vi "Write Paragraphe.vi"(8 "error in (no error)":errorcluster, 10 "Paragraphe cluster":T1, 11 "PDF Report Class in":refnum<class "PDF Report Class.lvclass">) -> (0 "error out":errorcluster, 3 "PDF Report Class out":refnum<class "PDF Report Class.lvclass">)   [LabVIEW 2019, in "PDF Report Class.lvclass"]
uses:
  <userlib>/Exaprom PDF/LV Class/PDF Report Class/PDF Report Class.lvclass
  <userlib>/Exaprom PDF/Controls/Initialization Controls/Defaut Paragraphe and Line Spacing.ctl
  <userlib>/Exaprom PDF/Controls/Text Controls/Texte alignement.ctl
  <userlib>/Exaprom PDF/Controls/Text Controls/Line spacing.ctl
  <userlib>/Exaprom PDF/LV Class/PDF Report Class/PDF Report Class.lvclass/PDF Report Class.ctl
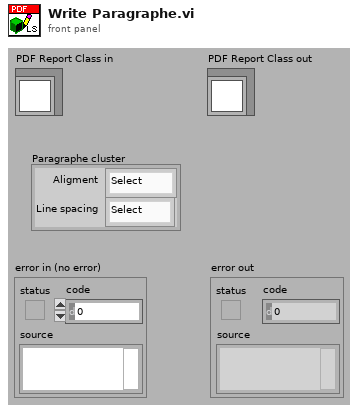
[diagram p1: front panel]
types:
  T1 = typedef "Defaut Paragraphe and Line Spacing.ctl" = cluster{" Aligment":T2, "Line spacing":T3}
  T2 = typedef "Texte alignement.ctl" = enum16{"Select", "CENTER", "JUSTIFY", "LEFT", "RIGHT"}
  T3 = typedef "Line spacing.ctl" = enum16{"Select", "1.0", "1.5", "2.0"}
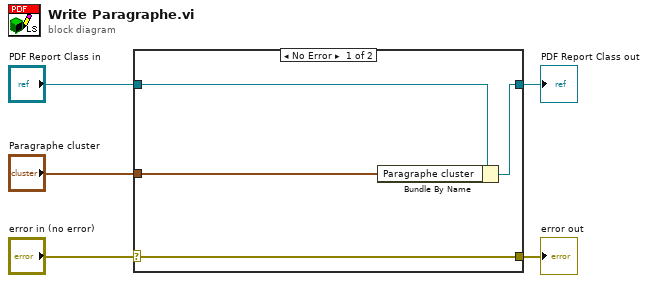
[diagram p0: block diagram]
diagram:
  n1 = case shown="No Error" "error in (no error)" {
    selector: "error in (no error)" -> [w9 w10]
    tunnel: [w9 w10] -> w4
    tunnel: [w7 w11] -> w2
    tunnel: "PDF Report Class in" -> [w8 w11]
    tunnel: "Paragraphe cluster" -> [w6 _]
    frame No Error {
      n2 = Bundle By Name(cluster=w8, "Paragraphe cluster"=w6) -> (w7:refnum<class "PDF Report Class.lvclass">)
    }
    frame Error {
    }
  }
  "error out" <- w4
  "PDF Report Class out" <- w2
